vi "svx_Orbit and Timebase Segment (N Ch - 1 Order).vi"(5 "reset? (F)":bool, 6 "end reach?":bool, 8 "error in (no error)":errorcluster, 9 "indice":cluster{"start":i32, "length":i32}, 11 "order data":dbl[][](array[numeric])) -> (0 "error out":errorcluster, 3 "order data out":dbl[][](array[numeric]))   [LabVIEW 2017]
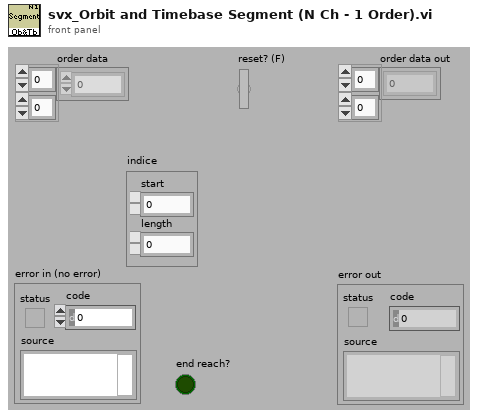
[diagram p1: front panel]
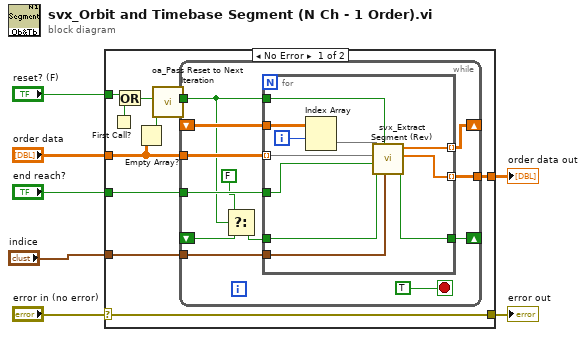
[diagram p0: block diagram]
diagram:
  n1 = case shown="No Error" "error in (no error)" {
    selector: "error in (no error)" -> [w14 w41]
    tunnel: "order data" -> [w12 _]
    tunnel: [w17 _] -> w6
    tunnel: "reset? (F)" -> [w16 _]
    tunnel: [w14 w41] -> w3
    tunnel: "indice" -> [w9 _]
    tunnel: "end reach?" -> [w8 _]
    frame No Error {
      n2 = First Call?() -> (First Call?: T/F=w15:bool)
      n3 = Or(x=w16, y=w15) -> (x .or. y?=w11:bool)
      n4 = Empty Array?(array=w12) -> (empty?=w13:bool)
      n5 = call <vilib>:"oa_Pass Reset to Next Iteration.vi"("trigger"=w13, "reset?(F)"=w11) -> ("reset out"=w10:bool)  [unwired: 9 in]
      n6 = while {
        tunnel: w12 -> [w28]
        shift-right: [w27] -> _
        shift-left: _ -> [w25]
        tunnel: w10 -> [w21]
        tunnel: [w26] -> w17
        tunnel: w9 -> [w24]
        shift-right: [w22] -> _
        shift-left: _ -> [w20]
        tunnel: w8 -> [w23]
        stop <- TRUE stop-if-true
        n7 = Select(t=FALSE, s=w21, f=w20) -> (s? t:f=w19:bool)
        n8 = for {
          tunnel: w28 -> [w38] mode=indexing
          tunnel: w25 -> [w40]
          tunnel: w21 -> [w36]
          tunnel: [w34] -> w27 mode=indexing
          tunnel: [w35] -> w26 mode=indexing
          tunnel: w24 -> [w33]
          tunnel: w23 -> [w32]
          tunnel: w19 -> [w31]
          tunnel: [w30] -> w22
          i -> [w39]
          n9 = Index Array(array=w40, index (row)=w39) -> (element=w37:dbl[])  [unwired: 1 in]
          n10 = call <vilib>:"svx_Extract Segment (Rev).vi"("indice"=w33, "reset?"=w36, "old end reached"=w31, "end reached"=w32, "data in"=w38, "old order data"=w37) -> ("end reached out"=w30:bool, "data out"=w35:dbl[], "remaining data"=w34:dbl[])  [unwired: 3 in]
        }
      }
    }
    frame Error {
    }
  }
  "order data out" <- w6
  "error out" <- w3
